vi "G_Bandas.vi"() -> ()   [LabVIEW 2020]
panel:
  out "Bandas":T1
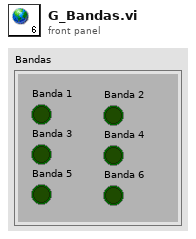
[diagram p1: front panel]
types:
  T1 = cluster{"Banda 1":bool, "Banda 2":bool, "Banda 3":bool, "Banda 4":bool, "Banda 5":bool, "Banda 6":bool}
diagram:
